vi "Write UI Ref Desc.vi"(8 "error in (no error)":errorcluster, 10 "UI Property":T1, 11 "UI Ref":refnum<vi>) -> (0 "error out":errorcluster)   [LabVIEW 2018, in "LF2R IDE.lvlib" / "LF2R IDE.lvclass"]
uses:
  LF2R IDE.lvclass
  Const UI Desc Property.ctl
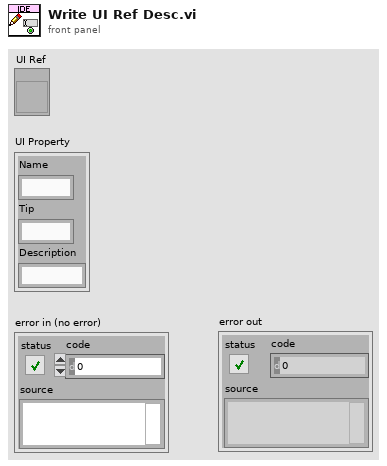
[diagram p1: front panel]
types:
  T1 = typedef "LF2R IDE.lvlib/LF2R IDE.lvclass/Const UI Desc Property.ctl" = cluster{"Name":string, "Tip":string, "Description":string}
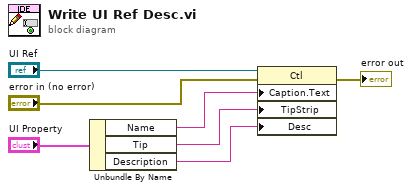
[diagram p0: block diagram]
diagram:
  n1 = Unbundle By Name("UI Property") -> ("Name"=w3:string, "Tip"=w2:string, "Description"=w1:string)
  n2 = property class="Ctl"(reference="UI Ref", error in="error in (no error)", "Caption.Text"=w3, "TipStrip"=w2, "Desc"=w1) -> (error out=→"error out":errorcluster)  [unwired: 1 out]
